vi "DB - [Config].[GeneralSetting].vi"(5 "Application":string, 7 "DB Connection":T2={"Open"=TRUE, "Close"=TRUE}, 8 "error in (no error)":errorcluster, 10 "[SettingId] Values":string[](array[string])=["GenericSystemId", "ScreenLockTimer"], 11 "connection reference":T1) -> (0 "SUMMARY":errorcluster, 2 "2D data":string[][](array[string]), 3 "connection reference":T1)   [LabVIEW 2013]
uses:
  <vilib>/addons/database/Connection.llb/Conn ObjectReference.ctl
  Controls/DB - OpenClose.ctl
  Controls/Global SRTRS.vi
  Controls/Global AMS.vi
  Controls/Global CMS.vi
  <vilib>/addons/database/Connection.llb/Conn Execute.vi
  <vilib>/addons/database/Recordset.llb/Rec Fetch Recordset Data (R).vi
  <vilib>/addons/database/Recordset.llb/Rec Destroy - Connection.vi
  <vilib>/addons/database/Connection.llb/DB Tools Open Connec (String).vi
  <vilib>/addons/database/_DB Variant To Data/Database Variant To Data.xnode
  <vilib>/addons/database/NI_Database_API.lvlib
panel:
  out "Close":errorcluster
  out "SQL Statement":string
  out "DB.Config.Setting":string="SRTRS.Config.Parameter"
  out "Connection Information":T3={"Connection "="SQL Server 32bit HPEnvy", "Username"="admin", "Password"="admin123"}
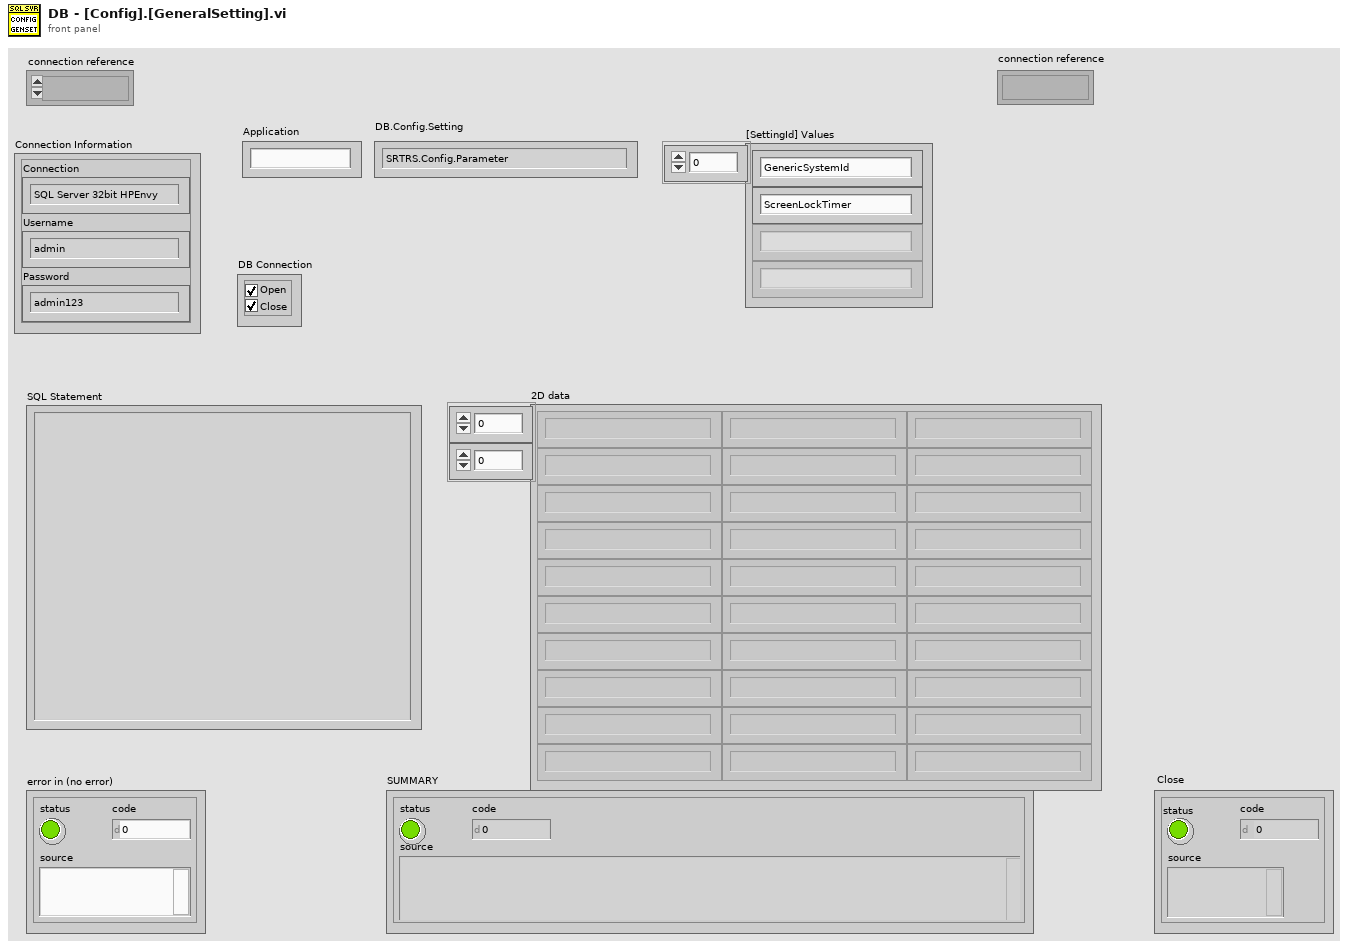
[diagram p1: front panel]
types:
  T1 = typedef "NI_Database_API.lvlib/Conn ObjectReference.ctl" = refnum<k1>
  T2 = typedef "DB - OpenClose.ctl" = cluster{"Open":bool, "Close":bool}
  T3 = cluster{"Connection ":string, "Username":string, "Password":string}
  T4 = typedef "Enum - InteractiveMode-SubVIMode.ctl" = enum16{"Interactive", "subVI Mode"}
  T5 = typedef "Connection Information Cluster.ctl" = cluster{"Connection ":string, "Username":string, "Password":string}
  T6 = typedef "DB - DB.Schema.Table.ctl" = cluster{"DB":string, "Schema":string, "Table":string}
  T7 = typedef "NI_Database_API.lvlib/Rec ObjectReference.ctl" = refnum<k1>
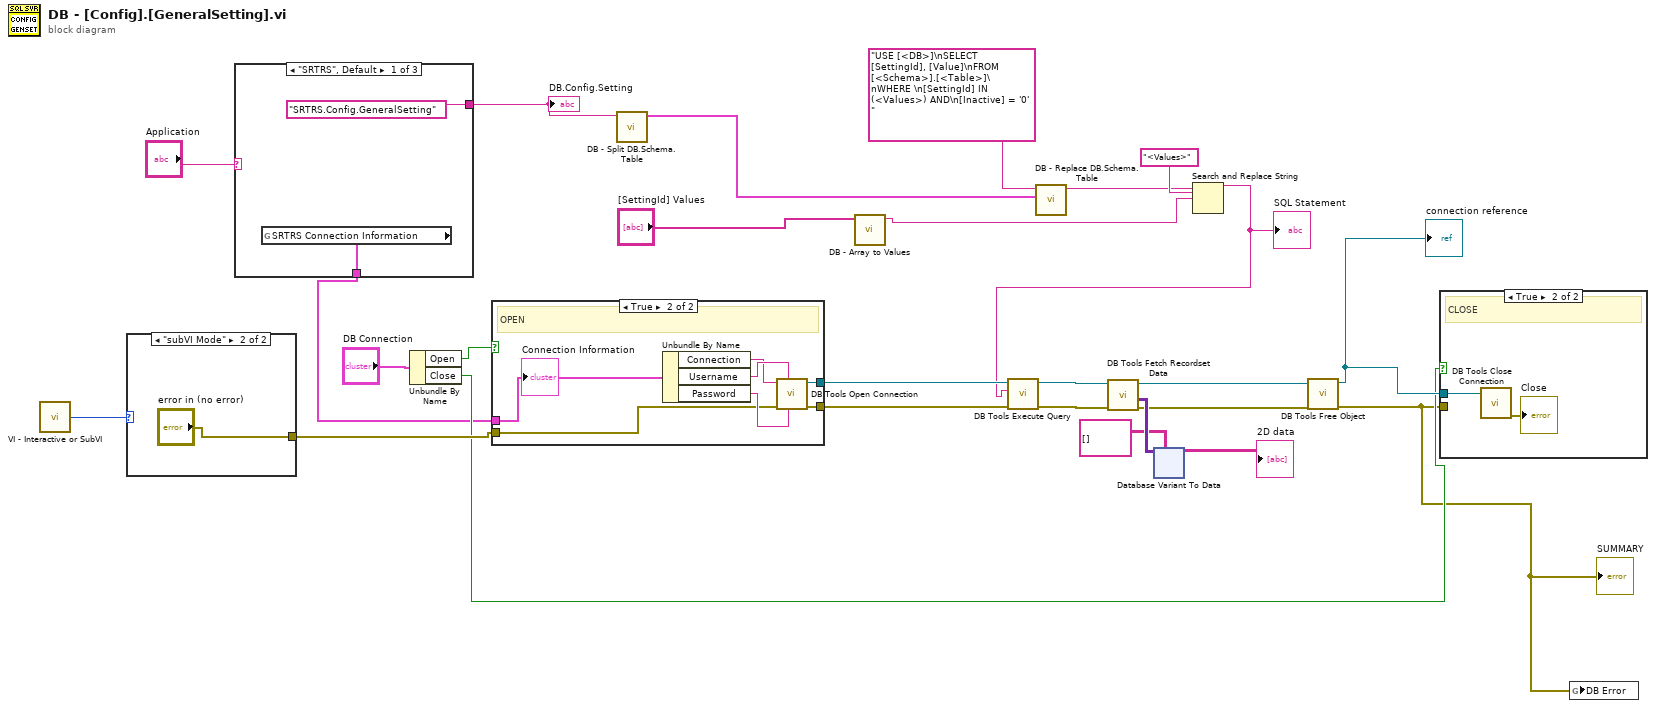
[diagram p0: block diagram]
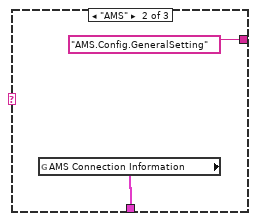
[diagram p2: hidden frame]
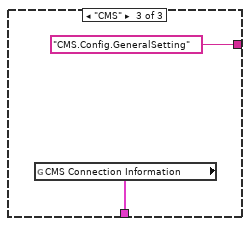
[diagram p3: hidden frame]
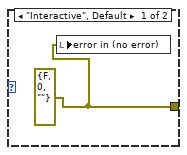
[diagram p5: hidden frame]
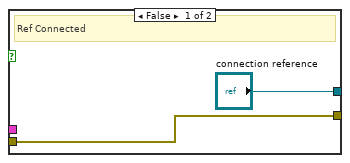
[diagram p6: hidden frame]
diagram:
  n1 = call "VI - Interactive or SubVI.vi"() -> ("Mode"=w24:T4)  [unwired: 5 in]
  n2 = case shown="\"subVI Mode\"" w24 {
    tunnel: [w27 "error in (no error)"] -> w23
    frame "Interactive", Default {
      w27 = errorcluster {"status"=FALSE, "code"=0, "source"=""} ("error in (no error)")
      n3 = local write "error in (no error)"(w27) -> ()
    }
    frame "subVI Mode" {
    }
  }
  n4 = case shown="\"SRTRS\", Default" "Application" {
    tunnel: ["SRTRS.Config.GeneralSetting" ("DB.Schema.Table\nSRTRS.Config.Parameter") "AMS.Config.GeneralSetting" ("DB.Schema.Table\nSRTRS.Config.Parameter") "CMS.Config.GeneralSetting" ("DB.Schema.Table\nSRTRS.Config.Parameter")] -> w7
    tunnel: [w29 w31 w33] -> w6
    frame "SRTRS", Default {
      n5 = global read "Global SRTRS.vi" "SRTRS Connection Information"() -> (w29:T5)
    }
    frame "AMS" {
      n6 = global read "Global AMS.vi" "AMS Connection Information"() -> (w31:T5)
    }
    frame "CMS" {
      n7 = global read "Global CMS.vi" "CMS Connection Information"() -> (w33:T5)
    }
  }
  "DB.Config.Setting" <- w7
  n8 = Unbundle By Name("DB Connection") -> ("Open"=w25:bool, "Close"=w13:bool)
  n9 = case shown="True" w25 {
    tunnel: ["connection reference" w40] -> w16
    tunnel: w23 -> [w35 w39]
    tunnel: [w35 w38] -> w15
    tunnel: w6 -> [_ w37]
    frame False {
      # "Ref Connected"
    }
    frame True {
      # "OPEN"
      n10 = Unbundle By Name(w37) -> ("Connection"=w42:string, "Username"=w43:string, "Password"=w41:string)
      n11 = call-poly <vilib>:"DB Tools Open Connection.vi"("password"=w41, "userID"=w43, "error in (no error)"=w39, "connection information"=w42) -> ("error out"=w38:errorcluster, "connection reference"=w40:T1)  [unwired: 4 in]
      "Connection Information" <- w37
    }
  }
  n12 = call "DB - Split DB.Schema.Table.vi"("DB.Schema.Table"=w7) -> ("DB.Schema.Table"=w12:T6)  [unwired: 10 in]
  n13 = call "DB - Array to Values.vi"("Array (0xFFFE autodetect)"="[SettingId] Values") -> ("<Values>"=w2:string)  [unwired: 10 in]
  n14 = call "DB - Replace DB.Schema.Table.vi"("DB.Schema.Table"=w12, "string in"="USE [<DB>]\nSELECT [SettingId], [Value]\nFROM [<Schema>].[<Table>]\nWHERE \n[SettingId] IN (<Values>) AND\n[Inactive] = '0' ") -> ("string out"=w1:string)  [unwired: 8 in, 1 out]
  n15 = Search and Replace String(input string=w1, search string="<Values>", replace string=w2) -> (result string=w4:string)  [unwired: 5 in, 3 out]
  "SQL Statement" <- w4
  n16 = call-poly <vilib>:"DB Tools Execute Query.vi"("error in (no error)"=w15, "SQL query"=w4, "connection reference"=w16) -> ("error out"=w22:errorcluster, "recordset reference"=w21:T7)  [unwired: 5 in]
  n17 = call-poly <vilib>:"DB Tools Fetch Recordset Data.vi"("error in (no error)"=w22, "recordset reference"=w21) -> ("error out"=w17:errorcluster, "recordset data"=w20:variant[][], "recordset reference out"=w18:T7)  [unwired: 3 in]
  n18 = xnode "Database Variant To Data"("database variant"=w20, "type"=string[][] []) -> ("data"=→"2D data":string[][])  [unwired: 1 in, 1 out]
  n19 = call-poly <vilib>:"DB Tools Free Object.vi"("error in (no error)"=w17, "recordset reference"=w18) -> ("error out"=w9:errorcluster, "connection reference"=w14:T1)  [unwired: 8 in]
  "SUMMARY" <- w9
  "connection reference" <- w14
  n20 = case shown="True" w13 {
    tunnel: w14 -> [_ w45]
    tunnel: w9 -> [_ _]
    frame False {
      # "Ref Connected"
    }
    frame True {
      # "CLOSE"
      n21 = call <vilib>:"DB Tools Close Connection.vi"("connection reference"=w45) -> ("error out"=→"Close":errorcluster)  [unwired: 6 in]
    }
  }
  n22 = global write "Global SRTRS.vi" "DB Error"(w9) -> ()
